vi "CD Import Export.vi"(8 "error in":errorcluster, 11 "Node Ptr":T1 format="%.0x") -> (0 "error out":errorcluster)   [LabVIEW 2017, in "PXImc System Explorer.lvlib"]
uses:
  PXImc System Explorer.lvlib
  <vilib>/NI Veristand/Custom Device API/Custom Device Item Ref.ctl
  <vilib>/NI VeriStand/Custom Device API/Custom Device API.lvlib
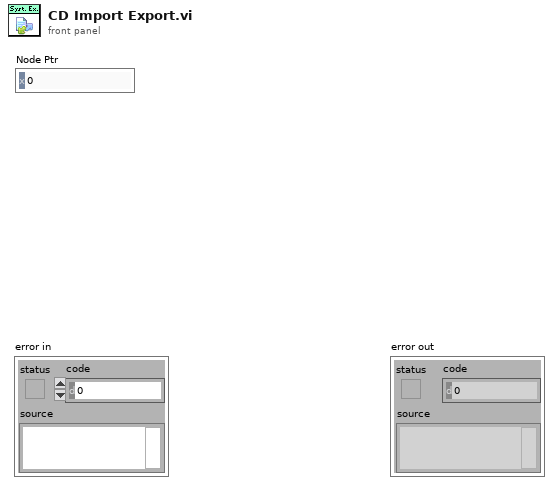
[diagram p1: front panel]
types:
  T1 = typedef "Custom Device API.lvlib/Custom Device Item Ref.ctl" = u64
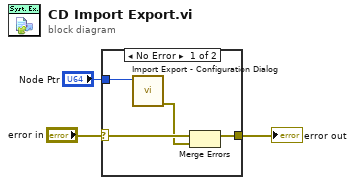
[diagram p0: block diagram]
diagram:
  n1 = case shown="No Error" "error in" {
    selector: "error in" -> [w7 w8]
    tunnel: [w5 w8] -> w2
    tunnel: "Node Ptr" -> [w6 _]
    frame No Error {
      n2 = call "Import Export - Configuration Dialog.vi"("Item Ref in"=w6) -> ("error out"=w4:errorcluster)  [unwired: 9 in, 1 out]
      n3 = Merge Errors(w7, w4) -> (w5:errorcluster)
    }
    frame Error {
    }
  }
  "error out" <- w2
